vi "Get Model Parameters - from SysDef.vi"(0 "System Definition Filepath (.nivssdf)":path, 11 "Error (in)":errorcluster) -> (4 "Models":string[](array[string]), 8 "Parameters":string[](array[string]), 15 "Error (out)":errorcluster)   [LabVIEW 2016]
uses:
  NationalInstruments.VeriStand.SystemDefinitionAPI
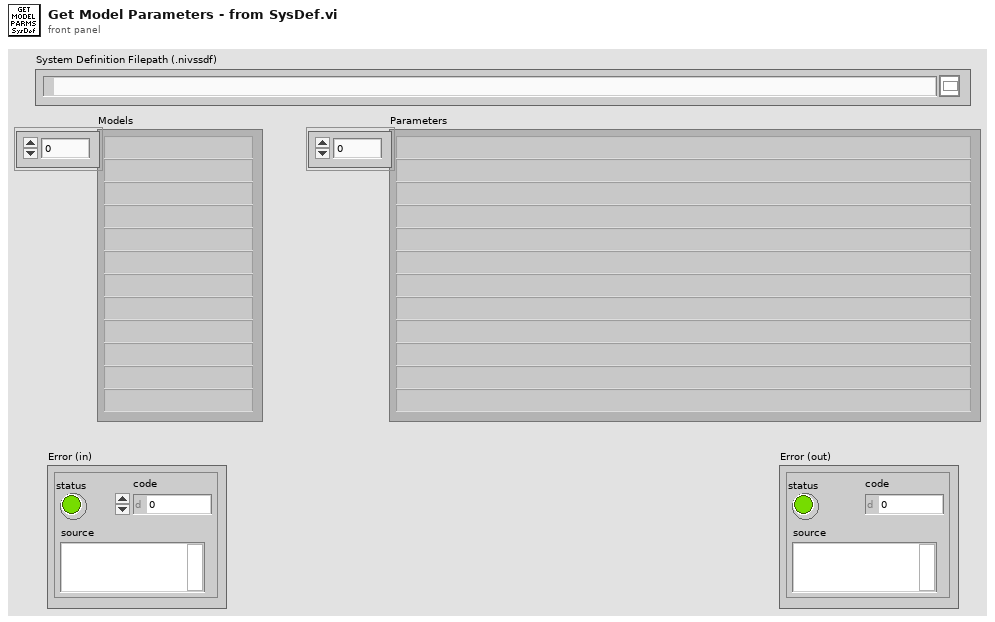
[diagram p1: front panel]
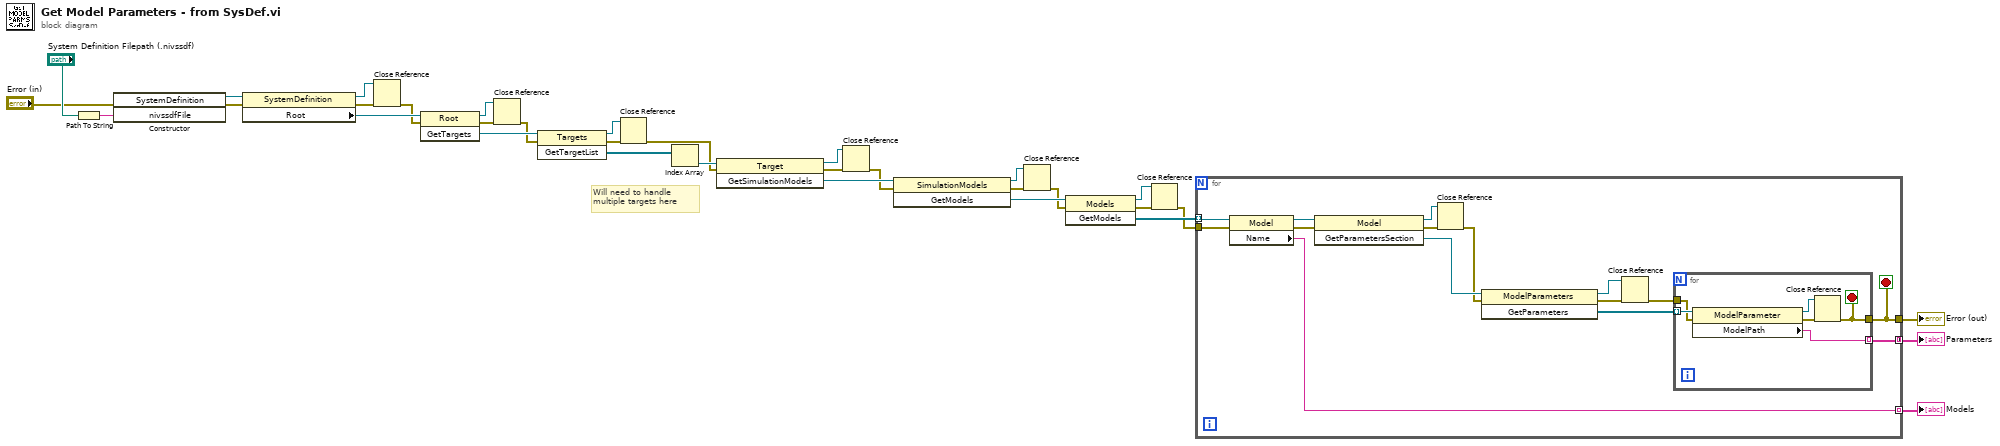
[diagram p0: block diagram]
diagram:
  # "Will need to handle multiple targets here"
  n1 = Path To String(path="System Definition Filepath (.nivssdf)") -> (string=w32:string)
  n2 = constructor class="SystemDefinition"(error in="Error (in)", "nivssdfFile"=w32) -> (reference out=w31:refnum<k24>, error out=w30:errorcluster)  [unwired: 2 in, 2 out]
  n3 = property class="SystemDefinition"(reference=w31, error in=w30) -> (reference out=w21:refnum<k24>, error out=w20:errorcluster, "Root"=w25:refnum<k24>)
  n4 = Close Reference(reference=w21, error in (no error)=w20) -> (error out=w19:errorcluster)
  n5 = invoke class="Root" method="GetTargets"(reference=w25, error in=w19) -> (reference out=w15:refnum<k24>, error out=w18:errorcluster, "GetTargets"=w24:refnum<k24>)  [unwired: 1 in]
  n6 = Close Reference(reference=w15, error in (no error)=w18) -> (error out=w17:errorcluster)
  n7 = invoke class="Targets" method="GetTargetList"(reference=w24, error in=w17) -> (reference out=w13:refnum<k24>, error out=w16:errorcluster, "GetTargetList"=w23:refnum<k24>[])  [unwired: 1 in]
  n8 = Close Reference(reference=w13, error in (no error)=w16) -> (error out=w14:errorcluster)
  n9 = Index Array(array=w23) -> (element=w29:refnum<k24>)  [unwired: 1 in]
  n10 = invoke class="Target" method="GetSimulationModels"(reference=w29, error in=w14) -> (reference out=w10:refnum<k24>, error out=w12:errorcluster, "GetSimulationModels"=w28:refnum<k24>)  [unwired: 1 in]
  n11 = Close Reference(reference=w10, error in (no error)=w12) -> (error out=w11:errorcluster)
  n12 = invoke class="SimulationModels" method="GetModels"(reference=w28, error in=w11) -> (reference out=w7:refnum<k24>, error out=w9:errorcluster, "GetModels"=w27:refnum<k24>)  [unwired: 1 in]
  n13 = Close Reference(reference=w7, error in (no error)=w9) -> (error out=w8:errorcluster)
  n14 = invoke class="Models" method="GetModels"(reference=w27, error in=w8) -> (reference out=w4:refnum<k24>, error out=w6:errorcluster, "GetModels"=w26:refnum<k24>[])  [unwired: 1 in]
  n15 = Close Reference(reference=w4, error in (no error)=w6) -> (error out=w5:errorcluster)
  n16 = for {
    tunnel: w26 -> [w47] mode=indexing
    tunnel: w5 -> [w48]
    tunnel: [w44] -> w22 mode=concatenating
    tunnel: [w35] -> w3 mode=indexing
    tunnel: [w34] -> w2
    stop <- w34 stop-if-true
    n17 = property class="Model"(reference=w47, error in=w48) -> (reference out=w42:refnum<k24>, error out=w43:errorcluster, "Name"=w35:string)
    n18 = invoke class="Model" method="GetParametersSection"(reference=w42, error in=w43) -> (reference out=w40:refnum<k24>, error out=w41:errorcluster, "GetParametersSection"=w46:refnum<k24>)  [unwired: 1 in]
    n19 = Close Reference(reference=w40, error in (no error)=w41) -> (error out=w39:errorcluster)
    n20 = invoke class="ModelParameters" method="GetParameters"(reference=w46, error in=w39) -> (reference out=w36:refnum<k24>, error out=w38:errorcluster, "GetParameters"=w45:refnum<k24>[])  [unwired: 1 in]
    n21 = Close Reference(reference=w36, error in (no error)=w38) -> (error out=w37:errorcluster)
    n22 = for {
      tunnel: w45 -> [w54] mode=indexing
      tunnel: [w49] -> w44 mode=indexing
      tunnel: w37 -> [w53]
      tunnel: [w51] -> w34
      stop <- w51 stop-if-true
      n23 = property class="ModelParameter"(reference=w54, error in=w53) -> (reference out=w50:refnum<k24>, error out=w52:errorcluster, "ModelPath"=w49:string)
      n24 = Close Reference(reference=w50, error in (no error)=w52) -> (error out=w51:errorcluster)
    }
  }
  "Models" <- w3
  "Error (out)" <- w2
  "Parameters" <- w22
